vi "Update.vi"(8 "error in (no error)":errorcluster, 11 "Level Controller in":refnum<class "Level Controller.lvclass">) -> (0 "error out":errorcluster, 3 "Level Controller out":refnum<class "Level Controller.lvclass">)   [LabVIEW 2012, in "Level Controller.lvlib" / "Level Controller.lvclass"]
uses:
  Level Controller.lvclass
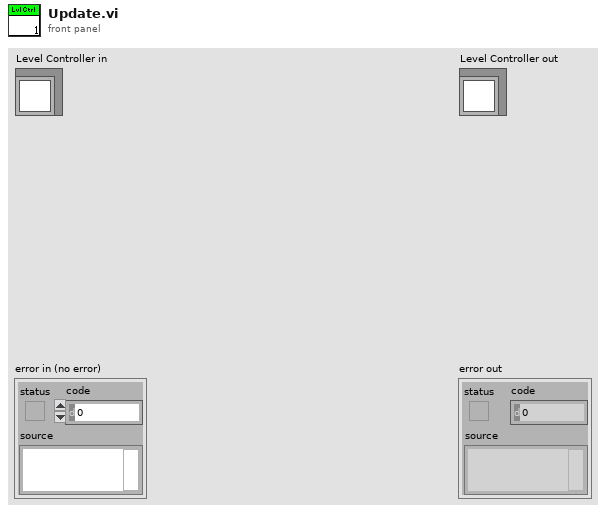
[diagram p1: front panel]
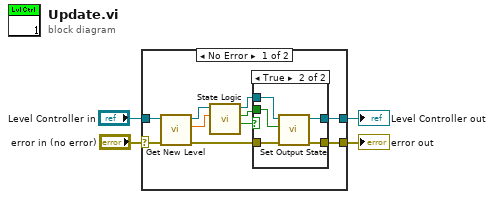
[diagram p0: block diagram]
diagram:
  n1 = case shown="No Error" "error in (no error)" {
    selector: "error in (no error)" -> [w13 w22]
    tunnel: "Level Controller in" -> [w14 w23]
    tunnel: [w7 w23] -> w2
    tunnel: [w5 w22] -> w1
    frame No Error {
      n2 = call-dynamic "Get New Level.vi"("error in (no error)"=w13, "Level Controller in"=w14) -> ("error out"=w6:errorcluster, "Level"=w11:dbl, "Level Controller out"=w12:refnum<class "Level Controller.lvclass">)  [unwired: 7 in]
      n3 = call "State Logic.vi"("Level"=w11, "Level Controller in"=w12) -> ("State Changed"=w10:bool, "Output State"=w8:bool, "Level Controller out"=w9:refnum<class "Level Controller.lvclass">)  [unwired: 7 in]
      n4 = case shown="True" w10 {
        tunnel: w9 -> [w16 w21]
        tunnel: w8 -> [_ w20]
        tunnel: [w16 w19] -> w7
        tunnel: w6 -> [w15 w18]
        tunnel: [w15 w17] -> w5
        frame False {
        }
        frame True {
          n5 = call-dynamic "Set Output State.vi"("error in (no error)"=w18, "Output State"=w20, "Level Controller in"=w21) -> ("error out"=w17:errorcluster, "Level Controller out"=w19:refnum<class "Level Controller.lvclass">)  [unwired: 7 in]
        }
      }
    }
    frame Error {
    }
  }
  "error out" <- w1
  "Level Controller out" <- w2
